vi "Stop DC_2_Coast.vi"(2 "DC Motors":T2={"DC Motor"=enum."DC Motor", "Address"=-1, "Address"=-1}, 3 "NXT":T3={"Hardware"="NXT", "Flattened String"=""}) -> (0 "NXT":T3={"Hardware"="NXT", "Flattened String"=""})   [LabVIEW 2010, in "4134Outputs.lvlib"]
uses:
  4134Outputs.lvlib
  <vilib>/NXT/Subs/LVHSConnector.ctl
  <vilib>/NXT/Subs/MotorXNode.DC Motor Type.ctl
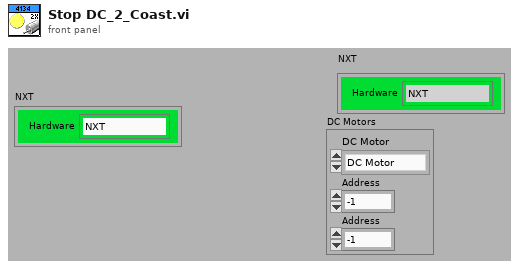
[diagram p1: front panel]
types:
  T1 = typedef "MotorXNode.DC Motor Type.ctl" = enum16{"DC Motor"}
  T2 = cluster{"DC Motor":T1, "Address":i16, "Address":i16}
  T3 = typedef "LVHSConnector.ctl" = cluster{"Hardware":string, "Flattened String":string}
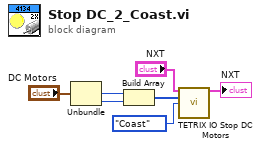
[diagram p0: block diagram]
diagram:
  n1 = Unbundle("DC Motors") -> ("Address"=w7:i16, "Address"=w5:i16)  [unwired: 1 out]
  n2 = Build Array(w7, w5) -> (w3:i16[])
  n3 = call <vilib>:"TETRIX IO Stop DC Motors.vi"("NXT"="NXT", "DC Motors"=w3, "Stopping Style"=enum16{"Coast", "Brake"}."Coast") -> ("NXT"=→"NXT":T3)  [unwired: 12 in]
